vi "ArrangeNodes SimulationSubVI.vi"(0 "varIn":T1={"nodes"=[], "edges"=[], "nodeSelected"=-1, "drag"=FALSE, "NodeRef"=[], "DragStart"={"X"=0, "Y"=0}, "fixedBeforeDrag"=FALSE, "Cancel"=FALSE, "ClassNodes"=[]} {"edges"."len" format="%.2f"; "nodes"."maxCornerDist" format="%.2f"; "nodes"."h" format="%.2f"; "nodes"."w" format="%.2f"; "nodes"."dy" format="%.2f"; "nodes"."dx" format="%.2f"; "nodes"."y" format="%.2f"; "nodes"."x" format="%.2f"}, 7 "AllowOverlap(False)":bool) -> (14 "varOut":T1={"nodes"=[], "edges"=[], "nodeSelected"=-1, "drag"=FALSE, "NodeRef"=[], "DragStart"={"X"=0, "Y"=0}, "fixedBeforeDrag"=FALSE, "Cancel"=FALSE, "ClassNodes"=[]} {"edges"."len" format="%.2f"; "nodes"."maxCornerDist" format="%.2f"; "nodes"."h" format="%.2f"; "nodes"."w" format="%.2f"; "nodes"."dy" format="%.2f"; "nodes"."dx" format="%.2f"; "nodes"."y" format="%.2f"; "nodes"."x" format="%.2f"})   [LabVIEW 2014]
uses:
  <resource>/Framework/Providers/Open_GDS/UML/ArrangeNodes/private/ArrangeNodes LocalVar.ctl
  <resource>/Framework/Providers/Open_GDS/UML/AbstractNode_class/AbstractNode.lvclass
  <resource>/Framework/Providers/Open_GDS/UML/General/Rectangle/Rectangle Rectangle2D.ctl
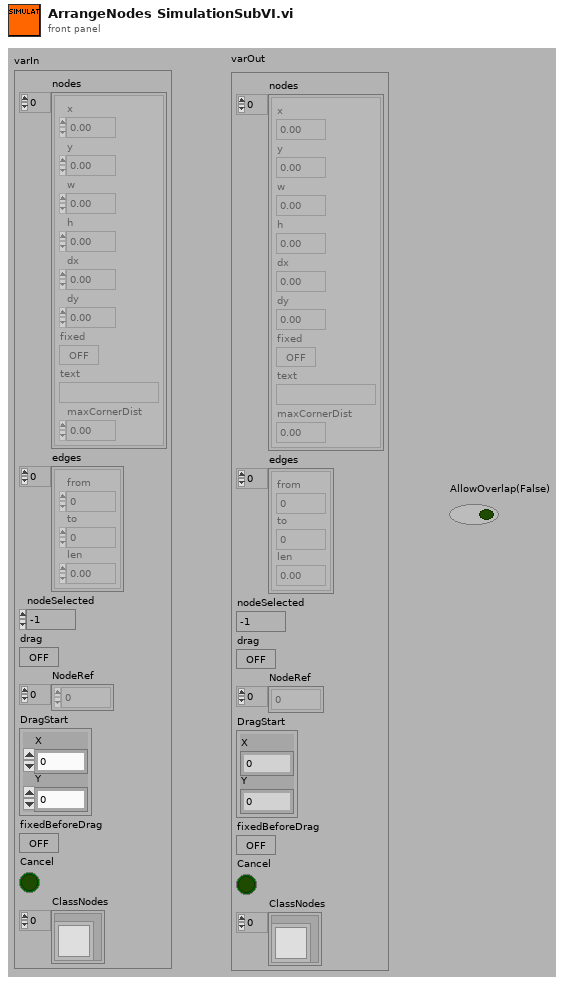
[diagram p1: front panel]
types:
  T1 = typedef "ArrangeNodes LocalVar.ctl" = cluster{"nodes":cluster{"x":dbl, "y":dbl, "w":dbl, "h":dbl, "dx":dbl, "dy":dbl, "fixed":bool, "text":string, "maxCornerDist":dbl}[], "edges":cluster{"from":i32, "to":i32, "len":dbl}[], "nodeSelected":i32, "drag":bool, "NodeRef":u32[], "DragStart":cluster{"X":i32, "Y":i32}, "fixedBeforeDrag":bool, "Cancel":bool, "ClassNodes":refnum<class "AbstractNode.lvclass">[]}
  T2 = cluster{"x":dbl, "y":dbl, "w":dbl, "h":dbl, "dx":dbl, "dy":dbl, "fixed":bool, "text":string, "maxCornerDist":dbl}[]
  T3 = cluster{"x":dbl, "y":dbl, "w":dbl, "h":dbl, "dx":dbl, "dy":dbl, "fixed":bool, "text":string, "maxCornerDist":dbl}
  T4 = typedef "Rectangle Rectangle2D.ctl" = cluster{"x":dbl, "y":dbl, "width":dbl, "height":dbl}
  T5 = typedef "Point Point2D.ctl" = cluster{"x":dbl, "y":dbl}
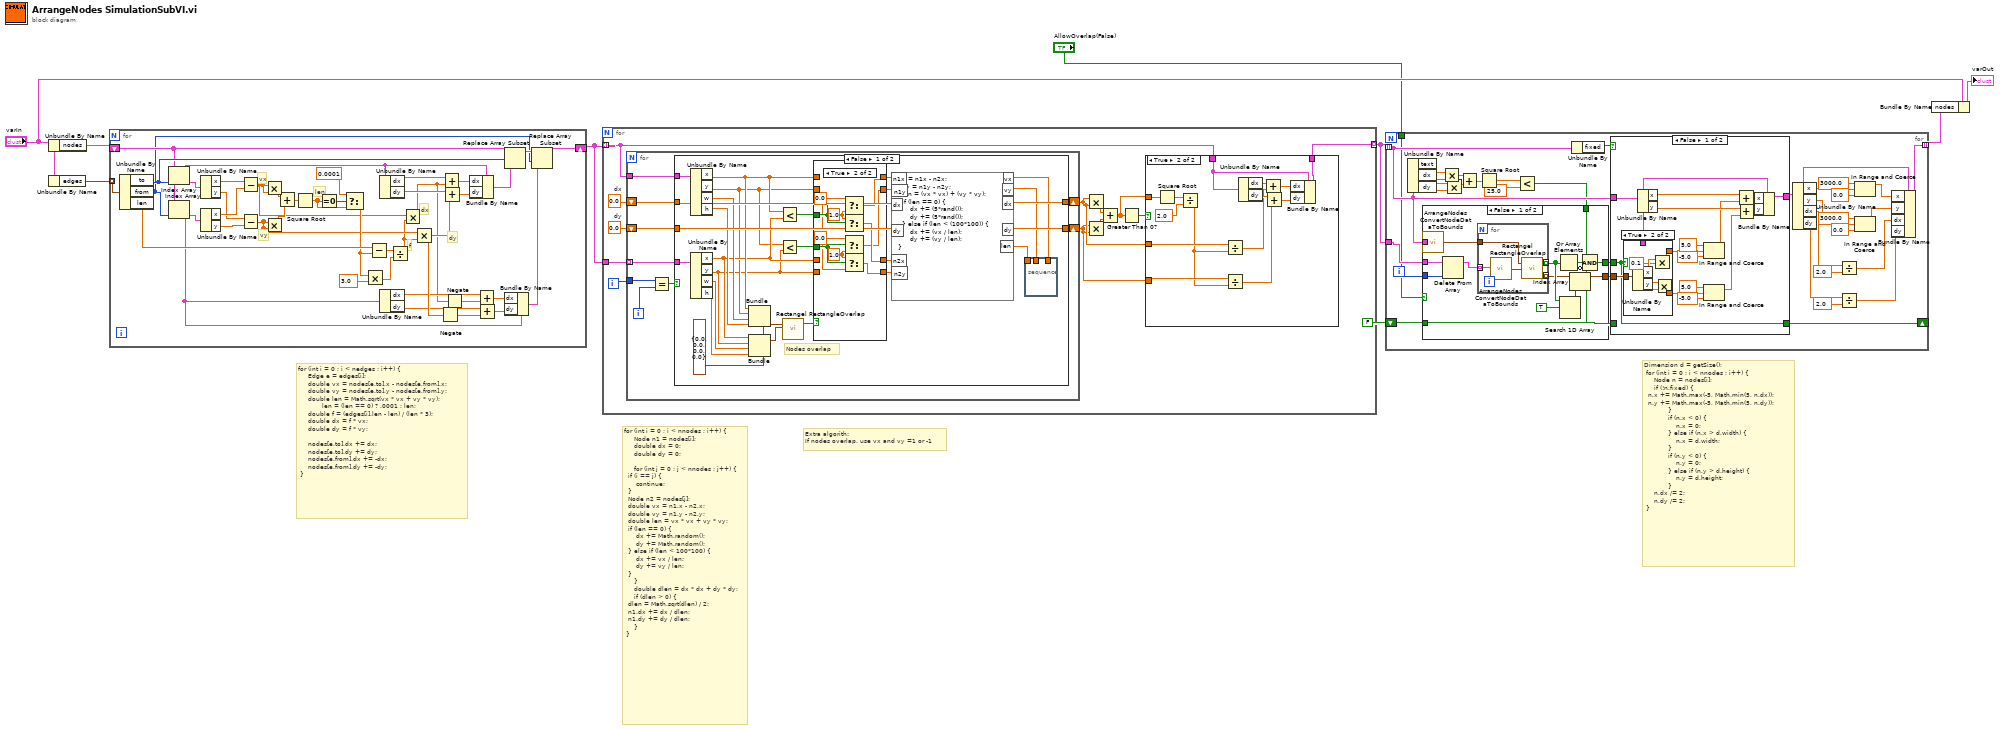
[diagram p0: block diagram]
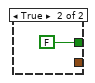
[diagram p2: hidden frame]
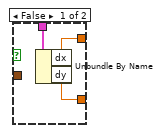
[diagram p3: hidden frame]
diagram:
  # "Extra algorith:\nIf nodes overlap, use vx and vy =1 or -1"
  # "Dimension d = getSize();\n\tfor (int i = 0 ; i < nnodes ; i++) {\n\t    Node n = nodes[i];\n\t    if (!n.fixed) {\n\t\tn.x += Math.max(-5, Math.min(5, n.dx));\n\t\tn.y += Math.max(-5, Math.min(5, n.dy));\n            }\n            if (n.x < 0) {\n                n.x = 0;\n            } else if (n.x > d.width) {\n                n.x = d.width;\n            }\n            if (n.y < 0) {\n                n.y = 0;\n            } else if (n.y > d.height) {\n                n.y = d.height;\n            }\n\t    n.dx /= 2;\n\t    n.dy /= 2;\n\t}"
  # "for (int i = 0 ; i < nnodes ; i++) {\n\t    Node n1 = nodes[i];\n\t    double dx = 0;\n\t    double dy = 0;\n\n\t    for (int j = 0 ; j < nnodes ; j++) {\n\t\tif (i == j) {\n\t\t    continue;\n\t\t}\n\t\tNode n2 = nodes[j];\n\t\tdouble vx = n1.x - n2.x;\n\t\tdouble vy = n1.y - n2.y;\n\t\tdouble len = vx * vx + vy * vy;\n\t\tif (len == 0) {\n\t\t    dx += Math.random();\n\t\t    dy += Math.random();\n\t\t} else if (len < 100*100) {\n\t\t    dx += vx / len;\n\t\t    dy += vy / len;\n\t\t}\n\t    }\n\t    double dlen = dx * dx + dy * dy;\n\t    if (dlen > 0) {\n\t\tdlen = Math.sqrt(dlen) / 2;\n\t\tn1.dx += dx / dlen;\n\t\tn1.dy += dy / dlen;\n\t    }\n\t}"
  # "for (int i = 0 ; i < nedges ; i++) {\n\t    Edge e = edges[i];\n\t    double vx = nodes[e.to].x - nodes[e.from].x;\n\t    double vy = nodes[e.to].y - nodes[e.from].y;\n\t    double len = Math.sqrt(vx * vx + vy * vy);\n            len = (len == 0) ? .0001 : len;\n\t    double f = (edges[i].len - len) / (len * 3);\n\t    double dx = f * vx;\n\t    double dy = f * vy;\n\n\t    nodes[e.to].dx += dx;\n\t    nodes[e.to].dy += dy;\n\t    nodes[e.from].dx += -dx;\n\t    nodes[e.from].dy += -dy;\n\t}"
  n1 = Unbundle By Name("varIn") -> ("nodes"=w8:T2)
  n2 = Unbundle By Name("varIn") -> ("edges"=w9:cluster{"from":i32, "to":i32, "len":dbl}[])
  n3 = for {
    tunnel: w9 -> [w49] mode=indexing
    shift-right: [w14] -> w4
    shift-left: w8 -> [w17]
    # "dy"
    # "dx"
    # "f"
    # "len"
    # "vy"
    # "vx"
    n4 = Unbundle By Name(w49) -> ("to"=w18:i32, "from"=w13:i32, "len"=w38:dbl)
    n5 = Index Array(array=w17, index=w18) -> (element=w33:T3)
    n6 = Index Array(array=w17, index=w13) -> (element=w19:T3)
    n7 = Unbundle By Name(w33) -> ("x"=w48:dbl, "y"=w45:dbl)
    n8 = Unbundle By Name(w19) -> ("x"=w47:dbl, "y"=w46:dbl)
    n9 = Subtract(x=w48, y=w47) -> (x-y=w28:dbl)
    n10 = Subtract(x=w45, y=w46) -> (x-y=w27:dbl)
    n11 = Multiply(x=w28, y=w28) -> (x*y=w43:dbl)
    n12 = Multiply(x=w27, y=w27) -> (x*y=w44:dbl)
    n13 = Add(x=w43, y=w44) -> (x+y=w42:dbl)
    n14 = Square Root(x=w42) -> (sqrt(x)=w39:dbl)
    n15 = Equal To 0?(x=w39) -> (x = 0?=w41:bool)
    n16 = Select(t=0.0001, s=w41, f=w39) -> (s? t:f=w36:dbl)
    n17 = Multiply(x=w36, y=3.0) -> (x*y=w34:dbl)
    n18 = Subtract(x=w38, y=w36) -> (x-y=w37:dbl)
    n19 = Unbundle By Name(w33) -> ("dx"=w32:dbl, "dy"=w31:dbl)
    n20 = Unbundle By Name(w19) -> ("dx"=w22:dbl, "dy"=w21:dbl)
    n21 = Divide(x=w37, y=w34) -> (x/y=w26:dbl)
    n22 = Multiply(x=w28, y=w26) -> (x*y=w20:dbl)
    n23 = Multiply(x=w27, y=w26) -> (x*y=w25:dbl)
    n24 = Negate(x=w25) -> (-x=w10:dbl)
    n25 = Add(x=w32, y=w20) -> (x+y=w30:dbl)
    n26 = Add(x=w31, y=w25) -> (x+y=w29:dbl)
    n27 = Negate(x=w20) -> (-x=w11:dbl)
    n28 = Bundle By Name(cluster=w33, "dx"=w30, "dy"=w29) -> (w16:T3)
    n29 = Add(x=w22, y=w11) -> (x+y=w23:dbl)
    n30 = Add(x=w21, y=w10) -> (x+y=w24:dbl)
    n31 = Replace Array Subset(array=w17, new element=w16, index=w18) -> (w15:T2)
    n32 = Bundle By Name(cluster=w19, "dx"=w23, "dy"=w24) -> (w12:T3)
    n33 = Replace Array Subset(array=w15, new element=w12, index=w13) -> (w14:T2)
  }
  n34 = for {
    tunnel: w4 -> [w50] mode=indexing
    tunnel: [w54] -> w3 mode=indexing
    tunnel: w4 -> [w51]
    i -> [w61]
    w60 = 0.0  # dx
    w59 = 0.0  # dy
    n35 = for {
      tunnel: w61 -> [w85]
      shift-right: [w82] -> w53
      shift-left: w60 -> [w81]
      shift-right: [w80] -> w52
      shift-left: w59 -> [w79]
      tunnel: w51 -> [w78] mode=indexing
      tunnel: w50 -> [w77]
      i -> [w84]
      n36 = Equal?(x=w85, y=w84) -> (x = y?=w83:bool)
      n37 = case shown="False" w83 {
        tunnel: [w108 w128] -> w82
        tunnel: w81 -> [w103 w128]
        tunnel: [w109 w127] -> w80
        tunnel: w79 -> [w110 w127]
        tunnel: w78 -> [w111 _]
        tunnel: w77 -> [w112 _]
        frame False {
          w104 = T4 {"x"=0.0, "y"=0.0, "width"=0.0, "height"=0.0} ("bounds2")
          # "Nodes overlap"
          n38 = Unbundle By Name(w112) -> ("x"=w91:dbl, "y"=w89:dbl, "w"=w102:dbl, "h"=w101:dbl)
          n39 = Unbundle By Name(w111) -> ("x"=w90:dbl, "y"=w88:dbl, "w"=w100:dbl, "h"=w99:dbl)
          n40 = Bundle(cluster=w104, "x"=w91, "y"=w89, "width"=w102, "height"=w101) -> (w98:T4)
          n41 = Bundle(cluster=w104, "x"=w90, "y"=w88, "width"=w100, "height"=w99) -> (w97:T4)
          n42 = Less?(x=w91, y=w90) -> (x < y?=w87:bool)
          n43 = Less?(x=w89, y=w88) -> (x < y?=w86:bool)
          n44 = call <resource>:"Rectangel RectangleOverlap.vi"("bounds1"=w98, "bounds2"=w97) -> ("overlap"=w96:bool)  [unwired: 2 in, 15 out]
          n45 = case shown="True" w96 {
            tunnel: w91 -> [w116 _]
            tunnel: w89 -> [w115 _]
            tunnel: w90 -> [w114 _]
            tunnel: w88 -> [w113 _]
            tunnel: [w116 w125] -> w95
            tunnel: [w115 w118] -> w94
            tunnel: [w114 w124] -> w93
            tunnel: [w113 w117] -> w92
            tunnel: w87 -> [_ w126]
            tunnel: w86 -> [_ w120]
            frame False {
            }
            frame True {
              w121 = 1.0 ("f")
              w119 = 0.0 ("t")
              w123 = 1.0 ("f")
              w122 = 0.0 ("t")
              n46 = Select(t=w122, s=w126, f=w123) -> (s? t:f=w125:dbl)
              n47 = Select(t=w123, s=w126, f=w122) -> (s? t:f=w124:dbl)
              n48 = Select(t=w119, s=w120, f=w121) -> (s? t:f=w118:dbl)
              n49 = Select(t=w121, s=w120, f=w119) -> (s? t:f=w117:dbl)
            }
          }
          n50 = formula code="vx = n1x - n2x;\n\t\tvy = n1y - n2y;\n\t\tlen = (vx * vx) + (vy * vy);\n\t\tif (len == 0) {\n\t\t    dx += (5*rand());\n\t\t    dy += (5*rand());\n\t\t} else if (len < (100*100)) {\n\t\t    dx += (vx / len);\n\t\t    dy += (vy / len);\n}"("n1x"=w95, "n1y"=w94, "n2x"=w93, "n2y"=w92, "dx"=w103, "dy"=w110) -> ("vx"=w105:dbl, "vy"=w106:dbl, "dx"=w108:dbl, "dy"=w109:dbl, "len"=w107:dbl)
          n51 = stacked-sequence {
            tunnel: w107 -> [_]
            tunnel: w106 -> [_]
            tunnel: w105 -> [_]
            frame #0 {
            }
          }
        }
        frame True {
          # "SKIP"
        }
      }
    }
    n52 = Multiply(x=w53, y=w53) -> (x*y=w58:dbl)
    n53 = Multiply(x=w52, y=w52) -> (x*y=w57:dbl)
    n54 = Add(x=w58, y=w57) -> (x+y=w55:dbl)
    n55 = Greater Than 0?(x=w55) -> (x > 0?=w56:bool)
    n56 = case shown="True" w56 {
      tunnel: w55 -> [_ w76]
      tunnel: w50 -> [w62 w69]
      tunnel: [w62 w68] -> w54
      tunnel: w53 -> [_ w67]
      tunnel: w52 -> [_ w66]
      frame False {
      }
      frame True {
        n57 = Square Root(x=w76) -> (sqrt(x)=w75:dbl)
        n58 = Divide(x=w75, y=2.0) -> (x/y=w65:dbl)
        n59 = Divide(x=w67, y=w65) -> (x/y=w64:dbl)
        n60 = Divide(x=w66, y=w65) -> (x/y=w63:dbl)
        n61 = Unbundle By Name(w69) -> ("dx"=w72:dbl, "dy"=w73:dbl)
        n62 = Add(x=w72, y=w64) -> (x+y=w71:dbl)
        n63 = Add(x=w73, y=w63) -> (x+y=w70:dbl)
        n64 = Bundle By Name(cluster=w69, "dx"=w71, "dy"=w70) -> (w68:T3)
      }
    }
  }
  n65 = for {
    tunnel: w3 -> [w138] mode=indexing
    tunnel: [w146] -> w5 mode=indexing
    tunnel: w3 -> [w145]
    shift-right: [w141] -> _
    shift-left: FALSE -> [w140]
    tunnel: "AllowOverlap(False)" -> [w129]
    i -> [w144]
    n66 = Unbundle By Name(w138) -> ("dx"=w137:dbl, "dy"=w136:dbl)  [unwired: 1 out]
    n67 = Multiply(x=w137, y=w137) -> (x*y=w135:dbl)
    n68 = Multiply(x=w136, y=w136) -> (x*y=w134:dbl)
    n69 = Add(x=w135, y=w134) -> (x+y=w133:dbl)
    n70 = Square Root(x=w133) -> (sqrt(x)=w130:dbl)
    n71 = Less?(x=w130, y=25.0 ("upper limit")) -> (x < y?=w131:bool)
    n72 = case shown="False" w129 {
      tunnel: w145 -> [w174 _]
      tunnel: w144 -> [w173 _]
      tunnel: [w167 _] -> w142
      tunnel: w140 -> [w166 _]
      tunnel: [w162 FALSE] -> w139
      tunnel: w138 -> [w164 _]
      tunnel: w131 -> [w163 _]
      frame False {
        n73 = call <resource>:"ArrangeNodes ConvertNodeDataToBounds.vi"("NodeData"=w164) -> ("NodeBounds"=w175:cluster{"x":dbl, "y":dbl, "w":dbl, "h":dbl})
        n74 = Delete From Array(array=w174, index=w173) -> (array with subset deleted=w172:T2)  [unwired: 1 in, 1 out]
        n75 = for {
          tunnel: w172 -> [w180] mode=indexing
          tunnel: w175 -> [w178]
          tunnel: [w177] -> w171 mode=indexing
          tunnel: [w176] -> w169 mode=indexing
          n76 = call <resource>:"ArrangeNodes ConvertNodeDataToBounds.vi"("NodeData"=w180) -> ("NodeBounds"=w179:cluster{"x":dbl, "y":dbl, "w":dbl, "h":dbl})
          n77 = call <resource>:"Rectangel RectangleOverlap.vi"("bounds1"=w178, "bounds2"=w179) -> ("overlap"=w177:bool, "translate1ToNotOverlap"=w176:T5)  [unwired: 2 in, 14 out]
        }
        n78 = Or Array Elements(Boolean array=w171) -> (logical OR=w165:bool)
        n79 = Search 1D Array(1D array=w171, element=TRUE) -> (index of element=w168:i32)  [unwired: 1 out]
        n80 = Index Array(array=w169, index=w168) -> (element=w167:T5)
        n81 = Compound Arithmetic op=AND(w163, w165, invert w166) -> (w162:bool)
      }
      frame True {
      }
    }
    n82 = Unbundle By Name(w138) -> ("fixed"=w143:bool)
    n83 = case shown="False" w143 {
      tunnel: w138 -> [w192 w208]
      tunnel: [w190 w208] -> w153
      tunnel: w139 -> [w182 _]
      tunnel: w142 -> [w183 _]
      tunnel: [w182 w207] -> w141
      tunnel: w140 -> [_ w207]
      frame False {
        n84 = case shown="True" w182 {
          tunnel: w192 -> [w200 _]
          tunnel: [w199 w203] -> w189
          tunnel: [w198 w201] -> w184
          tunnel: w183 -> [_ w206]
          frame False {
            n85 = Unbundle By Name(w200) -> ("dx"=w199:dbl, "dy"=w198:dbl)
          }
          frame True {
            w202 = 0.1 ("y")
            n86 = Unbundle By Name(w206) -> ("x"=w204:dbl, "y"=w205:dbl)
            n87 = Multiply(x=w204, y=w202) -> (x*y=w203:dbl)
            n88 = Multiply(x=w205, y=w202) -> (x*y=w201:dbl)
          }
        }
        n89 = Unbundle By Name(w192) -> ("x"=w195:dbl, "y"=w194:dbl)
        n90 = In Range and Coerce(upper limit=5.0, x=w189, lower limit=-5.0) -> (coerced(x)=w193:dbl)  [unwired: 1 out]
        n91 = In Range and Coerce(upper limit=5.0, x=w184, lower limit=-5.0) -> (coerced(x)=w191:dbl)  [unwired: 1 out]
        n92 = Add(x=w195, y=w193) -> (x+y=w196:dbl)
        n93 = Add(x=w194, y=w191) -> (x+y=w197:dbl)
        n94 = Bundle By Name(cluster=w192, "x"=w196, "y"=w197) -> (w190:T3)
      }
      frame True {
      }
    }
    n95 = Unbundle By Name(w153) -> ("x"=w161:dbl, "y"=w156:dbl, "dx"=w152:dbl, "dy"=w149:dbl)
    n96 = Divide(x=w152, y=2.0) -> (x/y=w147:dbl)
    n97 = Divide(x=w149, y=2.0) -> (x/y=w148:dbl)
    n98 = In Range and Coerce(upper limit=3000.0, x=w161, lower limit=0.0) -> (coerced(x)=w155:dbl)  [unwired: 1 out]
    n99 = In Range and Coerce(upper limit=3000.0, x=w156, lower limit=0.0) -> (coerced(x)=w154:dbl)  [unwired: 1 out]
    n100 = Bundle By Name(cluster=w153, "x"=w155, "y"=w154, "dx"=w147, "dy"=w148) -> (w146:T3)
  }
  n101 = Bundle By Name(cluster="varIn", "nodes"=w5) -> (→"varOut":T1)
